vi "FileIO_CopyFile.vi"(0 "Source Path":path, 1 "Target Path":path, 2 "Overwrite ?(F)":bool, 3 "Error In":errorcluster) -> (7 "New Path":path, 10 "Error Out":errorcluster)   [LabVIEW 2016]
doc: "This VI will copy a file from one directory to another. File will remain in old location as well as new location."
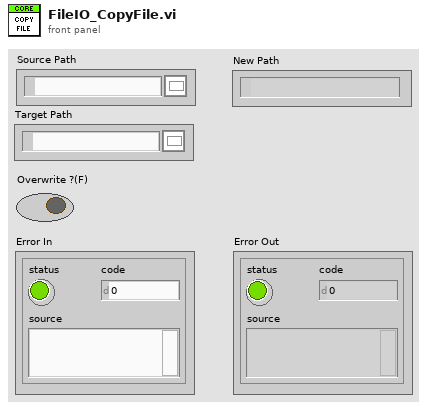
[diagram p1: front panel]
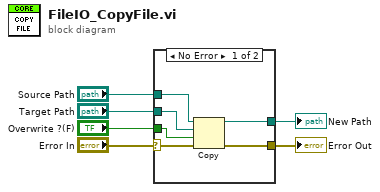
[diagram p0: block diagram]
diagram:
  n1 = case shown="No Error" "Error In" {
    selector: "Error In" -> [w12 w13]
    tunnel: "Target Path" -> [w10 _]
    tunnel: [w11 w13] -> w5
    tunnel: "Source Path" -> [w9 _]
    tunnel: [w8 _] -> w2
    tunnel: "Overwrite ?(F)" -> [w7 _]
    frame No Error {
      n2 = Copy(8:w12, 9:w7, 10:w10, 11:w9) -> (0:w11:errorcluster, 3:w8:path)  [unwired: 1 in, 1 out]
    }
    frame Error {
    }
  }
  "Error Out" <- w5
  "New Path" <- w2
